vi "Teleop.vi"(10 "Match Info":T1={"Autonomous Elapsed Seconds"=0.0, "TeleOp Elapsed Seconds"=0.0, "Disabled Elapsed Seconds"=0.0, "Visited Autonomous"=FALSE, "Visited TeleOp"=FALSE, "Visited Disabled"=FALSE, "Autonomous Settings"={"Autonomous Style"=enum."Independent", "VI Refnum"=refnum}}, 11 "Call Context":T2) -> ()   [LabVIEW 2017]
doc: "This VI is called for each TeleOp packet received from the DS where the robot is not disabled. It is often used to read from the joysticks and update I/O or to update setpoints for timed control loops. It should complete and return within 20 milliseconds or it may miss DS packets."
uses:
  <vilib>/Rock Robotics/WPI/DriverStation/WPI_DriverStationDerivedRobotMode.ctl
  <vilib>/Rock Robotics/WPI/DriverStation/WPI_DriverStationMatch Info.ctl
  <vilib>/Rock Robotics/WPI/Relay/WPI_RelayValue.ctl
  <vilib>/Rock Robotics/WPI/Utilities/WPI_GetSetVariantRefNum.vi
  <vilib>/Rock Robotics/Network Tables/NT Write Boolean Array.vi
  <vilib>/Rock Robotics/Network Tables/NT Write Numeric Array.vi
  <vilib>/Rock Robotics/Network Tables/NT Read Boolean.vi
  <vilib>/Rock Robotics/Network Tables/NT Read Number.vi
  Robot Global Data.vi
  <vilib>/Rock Robotics/Network Tables/NT Write Number.vi
panel:
  out "Sample Slider 0":dbl(slide) scale=0.0..5.0
  out "Sample Boolean 1":bool
  out "Sample Boolean 0":bool
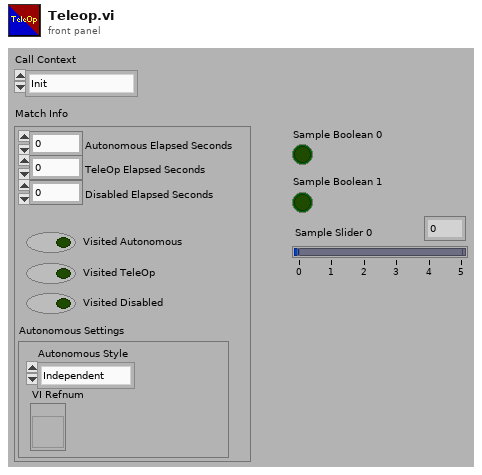
[diagram p1: front panel]
types:
  T1 = typedef "WPI_DriverStationMatch Info.ctl" = cluster{"Autonomous Elapsed Seconds":dbl, "TeleOp Elapsed Seconds":dbl, "Disabled Elapsed Seconds":dbl, "Visited Autonomous":bool, "Visited TeleOp":bool, "Visited Disabled":bool, "Autonomous Settings":cluster{"Autonomous Style":enum16{"Iterative", "Independent"}, "VI Refnum":refnum<vi>}}
  T2 = typedef "WPI_DriverStationDerivedRobotMode.ctl" = enum16{"Init", "Execute", "Stop"}
  T3 = typedef "WPI_RobotDriveDevRef.ctl" = cluster{"DevStatus":errorcluster, "Motors[]":T4[], "Square Inputs":bool, "Max Output":dbl}
  T4 = typedef "WPI_MotorControlDeviceRef.ctl" = cluster{"DeviceStatus":errorcluster, "Type":T5, "PWM":cluster{"PWM Channel":T6, "DeadBand":T7}, "CAN":cluster{"Device Number":u8, "SetOutput VI Ref":variant, "GetOutput VI Ref":variant, "Enable VI Ref":variant, "Disable VI Ref":variant, "Data":variant}, "Invert":bool, "DIO PWM":cluster{"PWM \"Enable\" Channel":T6, "DIOChannel":T8, "PWM Rate":dbl}}
  T5 = typedef "WPI_MotorControlType.ctl" = enum16{"PWM", "CAN", "DIO PWM"}
  T6 = typedef "FPGA_DIOPWMChannel.ctl" = enum8{"PWM 0", "PWM 1", "PWM 2", "PWM 3", "PWM 4", "PWM 5", "PWM 6", "PWM 7", "PWM 8", "PWM 9", "PWM MXP 0", "PWM MXP 1", "PWM MXP 2", "PWM MXP 3", "PWM MXP 4", "PWM MXP 5", "PWM MXP 6", "PWM MXP 7", "PWM MXP 8", "PWM MXP 9", "Invalid"}
  T7 = typedef "WPI_PWMDeadband.ctl" = cluster{"Name":string, "maxPositivePwm":i32, "minPositivePwm":i32, "centerPwm":i32, "maxNegativePwm":i32, "minNegativePwm":i32, "angularRange":u16}
  T8 = typedef "FPGA_DIOChannel.ctl" = enum8{"DIO 0", "DIO 1", "DIO 2", "DIO 3", "DIO 4", "DIO 5", "DIO 6", "DIO 7", "DIO 8", "DIO 9", "DIO MXP 0", "DIO MXP 1", "DIO MXP 2", "DIO MXP 3", "DIO MXP 4", "DIO MXP 5", "DIO MXP 6", "DIO MXP 7", "DIO MXP 8", "DIO MXP 9", "DIO MXP 10", "DIO MXP 11", "DIO MXP 12", "DIO MXP 13", "DIO MXP 14", "DIO MXP 15", "SPI Port CS1", "SPI Port CS2", "SPI Port CS3", "SPI Port MISO", "SPI Port MOSI", "Invalid"}
  T9 = typedef "WPI_JoystickDevRef.ctl" = cluster{"Device":T10}
  T10 = typedef "WPI_JoystickDeviceEnum.ctl" = enum16{"USB 0", "USB 1", "USB 2", "USB 3", "USB 4", "USB 5"}
  T11 = typedef "WPI_RelayValue.ctl" = enum16{"Off", "On", "Forward", "Reverse"}
  T12 = typedef "WPI_RelayDevRef.ctl" = cluster{"DevStatus":errorcluster, "Relay Channel":T13, "Relay Direction":T14}
  T13 = typedef "FPGA_DIORelayChannel.ctl" = enum8{"Relay 0", "Relay 1", "Relay 2", "Relay 3", "Invalid"}
  T14 = typedef "WPI_RelayDirection.ctl" = enum16{"Both directions", "Forward only", "Reverse only"}
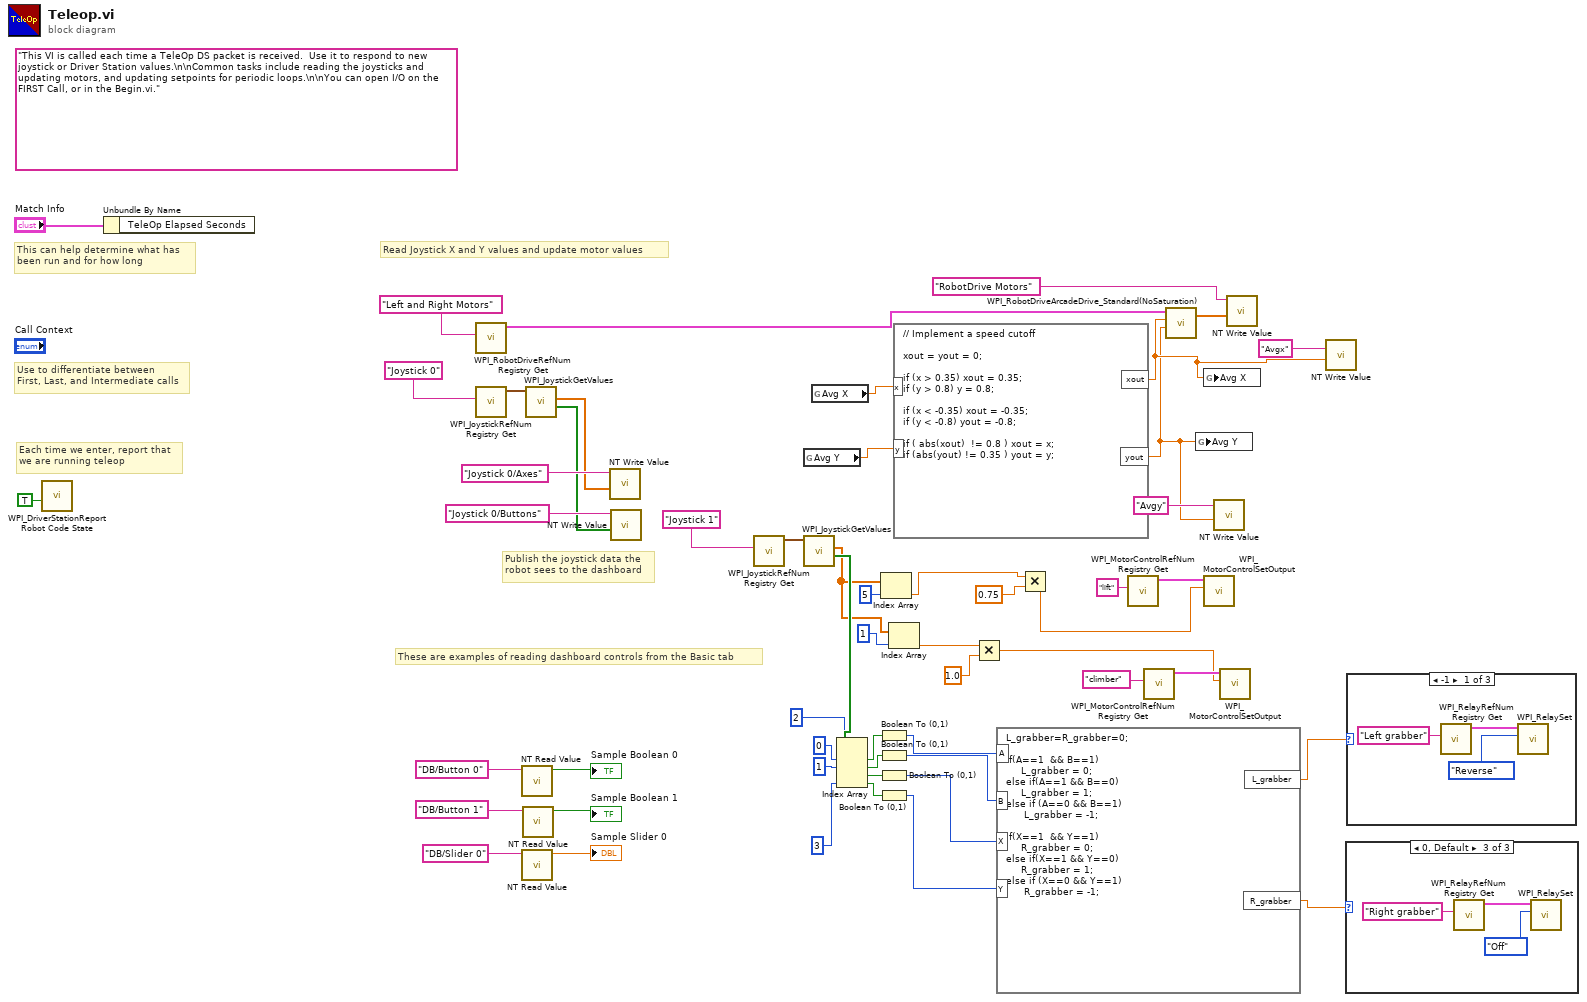
[diagram p0: block diagram]
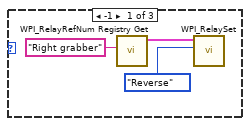
[diagram p2: hidden frame]
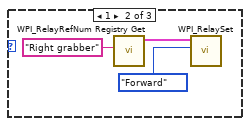
[diagram p3: hidden frame]
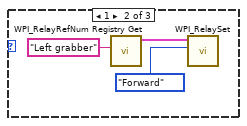
[diagram p4: hidden frame]
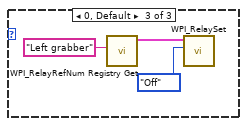
[diagram p5: hidden frame]
diagram:
  (unwired) "This VI is called each time a TeleOp DS packet is received.  Use it to respond to new joystick or Driver Station values.\n\nCommon tasks include reading the joysticks and updating motors, and updating setpoints for periodic loops.\n\nYou can open I/O on the FIRST Call, or in the Begin.vi."
  # "These are examples of reading dashboard controls from the Basic tab"
  # "Publish the joystick data the\nrobot sees to the dashboard"
  # "Each time we enter, report that\nwe are running teleop"
  # "Use to differentiate between\nFirst, Last, and Intermediate calls"
  # "This can help determine what has\nbeen run and for how long"
  # "Read Joystick X and Y values and update motor values"
  n1 = call <vilib>:"WPI_DriverStationReport Robot Code State.vi"("TeleOp"=TRUE ("Autonomous")) -> ()  [unwired: 10 in, 1 out]
  n2 = Unbundle By Name("Match Info") -> ()  [unwired: 1 out]
  n3 = call <vilib>:"WPI_RobotDriveRefNum Registry Get.vi"("refnum name"="Left and Right Motors") -> ("RobotDriveDevRef"=w37:T3)  [unwired: 1 in, 9 out]
  n4 = call <vilib>:"WPI_JoystickRefNum Registry Get.vi"("refnum name"="Joystick 0") -> ("JoystickDevRef"=w51:T9)  [unwired: 1 in, 9 out]
  n5 = call-poly <vilib>:"NT Read Value.vi"("Name"="DB/Button 0" ("refnum name")) -> ("Boolean"=→"Sample Boolean 0":bool)  [unwired: 9 in, 1 out]
  n6 = call-poly <vilib>:"NT Read Value.vi"("Name"="DB/Slider 0" ("refnum name")) -> ("Numeric"=→"Sample Slider 0":dbl)  [unwired: 9 in, 1 out]
  n7 = call-poly <vilib>:"NT Read Value.vi"("Name"="DB/Button 1" ("refnum name")) -> ("Boolean"=→"Sample Boolean 1":bool)  [unwired: 9 in, 1 out]
  n8 = call <vilib>:"WPI_JoystickGetValues.vi"("JoystickDevRef"=w51) -> ("Buttons"=w46:bool[], "Axes"=w47:dbl[])  [unwired: 6 in, 3 out]
  n9 = call-poly <vilib>:"NT Write Value.vi"("Numeric Array"=w47, "Name"="Joystick 0/Axes") -> ()  [unwired: 9 in, 1 out]
  n10 = call-poly <vilib>:"NT Write Value.vi"("Boolean Array"=w46, "Name"="Joystick 0/Buttons") -> ()  [unwired: 9 in, 1 out]
  n11 = call <vilib>:"WPI_JoystickRefNum Registry Get.vi"("refnum name"="Joystick 1") -> ("JoystickDevRef"=w25:T9)  [unwired: 1 in, 9 out]
  n12 = global read "Robot Global Data.vi" "Avg Y"() -> (w35:dbl)
  n13 = call <vilib>:"WPI_JoystickGetValues.vi"("JoystickDevRef"=w25) -> ("Buttons"=w22:bool[], "Axes"=w8:dbl[])  [unwired: 6 in, 3 out]
  n14 = global read "Robot Global Data.vi" "Avg X"() -> (w36:dbl)
  n15 = Index Array(array=w22, index #1=0 ("index"), index #2=1 ("index"), index #3=2 ("index"), index #4=3 ("index")) -> (element #1=w17:bool, element #2=w13:bool, element #3=w14:bool, element #4=w15:bool)
  n16 = Boolean To (0,1)(Boolean=w17) -> (0, 1=w16:i16)
  n17 = Boolean To (0,1)(Boolean=w13) -> (0, 1=w12:i16)
  n18 = Boolean To (0,1)(Boolean=w14) -> (0, 1=w11:i16)
  n19 = Boolean To (0,1)(Boolean=w15) -> (0, 1=w10:i16)
  n20 = Index Array(array=w8, index=5) -> (element=w23:dbl)
  n21 = Index Array(array=w8, index=1) -> (element=w6:dbl)
  n22 = formula code="// Implement a speed cutoff\n\nxout = yout = 0;\n\nif (x > 0.35) xout = 0.35; \nif (y > 0.8) y = 0.8;\n\nif (x < -0.35) xout = -0.35;\nif (y < -0.8) yout = -0.8;\n\nif ( abs(xout)  != 0.8 ) xout = x;\nif (abs(yout) != 0.35 ) yout = y;"("x"=w36, "y"=w35) -> ("xout"=w33:dbl, "yout"=w31:dbl)
  n23 = Multiply(x=w6, y=1.0) -> (x*y=w3:dbl)
  n24 = formula code="L_grabber=R_grabber=0;\n\nif(A==1  && B==1)\n     L_grabber = 0;\nelse if(A==1 && B==0)\n     L_grabber = 1;\nelse if (A==0 && B==1)\n      L_grabber = -1;\n\nif(X==1  && Y==1)\n     R_grabber = 0;\nelse if(X==1 && Y==0)\n     R_grabber = 1;\nelse if (X==0 && Y==1)\n      R_grabber = -1;"("A"=w16, "B"=w12, "X"=w11, "Y"=w10) -> ("L_grabber"=w2:dbl, "R_grabber"=w1:dbl)
  n25 = Multiply(x=w23, y=0.75) -> (x*y=w27:dbl)
  n26 = call <vilib>:"WPI_MotorControlRefNum Registry Get.vi"("refnum name"="lift") -> ("MotorControlDevRef"=w29:T4)  [unwired: 9 in, 1 out]
  n27 = call <vilib>:"WPI_MotorControlRefNum Registry Get.vi"("refnum name"="climber") -> ("MotorControlDevRef"=w4:T4)  [unwired: 9 in, 1 out]
  n28 = call <vilib>:"WPI_RobotDriveArcadeDrive_Standard(NoSaturation).vi"("Y axis value"=w31, "X axis value"=w33, "RobotDriveDevRef"=w37) -> ("Motor Values"=w38:dbl[])  [unwired: 1 in, 7 out]
  n29 = global write "Robot Global Data.vi" "Avg Y"(w31) -> ()
  n30 = global write "Robot Global Data.vi" "Avg X"(w33) -> ()
  n31 = call <vilib>:"WPI_MotorControlSetOutput.vi"("Output"=w27, "MotorControlDevRef"=w29) -> ()  [unwired: 7 in, 3 out]
  n32 = call-poly <vilib>:"NT Write Value.vi"("Numeric"=w31, "Name"="Avgy") -> ()  [unwired: 9 in, 1 out]
  n33 = call <vilib>:"WPI_MotorControlSetOutput.vi"("Output"=w3, "MotorControlDevRef"=w4) -> ()  [unwired: 7 in, 3 out]
  n34 = call-poly <vilib>:"NT Write Value.vi"("Numeric Array"=w38, "Name"="RobotDrive Motors") -> ()  [unwired: 9 in, 1 out]
  n35 = call-poly <vilib>:"NT Write Value.vi"("Numeric"=w33, "Name"="Avgx") -> ()  [unwired: 9 in, 1 out]
  n36 = case shown="0, Default" w1 {
    frame -1 {
      n37 = call <vilib>:"WPI_RelayRefNum Registry Get.vi"("refnum name"="Right grabber") -> ("RelayDevRef"=w57:T12)  [unwired: 9 in, 1 out]
      n38 = call <vilib>:"WPI_RelaySet.vi"("RelayValue"=WPI_RelayValue."Reverse", "RelayDevRef"=w57) -> ()  [unwired: 8 in, 2 out]
    }
    frame 1 {
      n39 = call <vilib>:"WPI_RelayRefNum Registry Get.vi"("refnum name"="Right grabber") -> ("RelayDevRef"=w60:T12)  [unwired: 9 in, 1 out]
      n40 = call <vilib>:"WPI_RelaySet.vi"("RelayValue"=WPI_RelayValue."Forward", "RelayDevRef"=w60) -> ()  [unwired: 8 in, 2 out]
    }
    frame 0, Default {
      n41 = call <vilib>:"WPI_RelayRefNum Registry Get.vi"("refnum name"="Right grabber") -> ("RelayDevRef"=w62:T12)  [unwired: 9 in, 1 out]
      n42 = call <vilib>:"WPI_RelaySet.vi"("RelayValue"=WPI_RelayValue."Off", "RelayDevRef"=w62) -> ()  [unwired: 8 in, 2 out]
    }
  }
  n43 = case shown="-1" w2 {
    frame -1 {
      n44 = call <vilib>:"WPI_RelayRefNum Registry Get.vi"("refnum name"="Left grabber") -> ("RelayDevRef"=w66:T12)  [unwired: 9 in, 1 out]
      n45 = call <vilib>:"WPI_RelaySet.vi"("RelayValue"=WPI_RelayValue."Reverse", "RelayDevRef"=w66) -> ()  [unwired: 8 in, 2 out]
    }
    frame 1 {
      n46 = call <vilib>:"WPI_RelayRefNum Registry Get.vi"("refnum name"="Left grabber") -> ("RelayDevRef"=w69:T12)  [unwired: 9 in, 1 out]
      n47 = call <vilib>:"WPI_RelaySet.vi"("RelayValue"=WPI_RelayValue."Forward", "RelayDevRef"=w69) -> ()  [unwired: 8 in, 2 out]
    }
    frame 0, Default {
      n48 = call <vilib>:"WPI_RelayRefNum Registry Get.vi"("refnum name"="Left grabber") -> ("RelayDevRef"=w71:T12)  [unwired: 9 in, 1 out]
      n49 = call <vilib>:"WPI_RelaySet.vi"("RelayValue"=WPI_RelayValue."Off", "RelayDevRef"=w71) -> ()  [unwired: 8 in, 2 out]
    }
  }
